vi "AudioTest.AudioTestUtil, Read Config.vi"(7 "File":path=path "c:/MTE/Audio Test/Config/Audio Util Config.ini", 8 "RtSetup":T1={"Play Device"="Utah", "Play Volume"=80.0, "DTMF Channel"=7, "Rec Device"="Jabra"} caption="Right Speaker Test Setup", 9 "LftSetup":T1={"Play Device"="Utah", "Play Volume"=80.0, "DTMF Channel"=4, "Rec Device"="Jabra"} caption="Left Speaker Test Setup", 10 "MicSetup":T1={"Play Device"="Jabra", "Play Volume"=60.0, "DTMF Channel"=1, "Rec Device"="Valve"} caption="Microphone Test Setup", 11 "ToneDur":dbl=0.3 caption="Tone Duration(s)") -> (0 "RtSetup Out":T1={"Play Device"="Utah", "Play Volume"=80.0, "DTMF Channel"=7, "Rec Device"="Jabra"} caption="Right Speaker Test Setup", 1 "LftSetup Out":T1={"Play Device"="Utah", "Play Volume"=80.0, "DTMF Channel"=4, "Rec Device"="Jabra"} caption="Left Speaker Test Setup", 2 "MicSetup Out":T1={"Play Device"="Jabra", "Play Volume"=60.0, "DTMF Channel"=1, "Rec Device"="Valve"} caption="Microphone Test Setup", 3 "ToneDur Out":dbl=0.3 caption="Tone Duration(s)", 4 "error out":errorcluster)   [LabVIEW 2018]
uses:
  <vilib>/Utility/config.llb/Read Key (Double).vi
  <vilib>/Utility/config.llb/Read Key (String).vi
  <vilib>/Utility/config.llb/Read Key (I32).vi
  <vilib>/Utility/config.llb/NI_LVConfig.lvlib
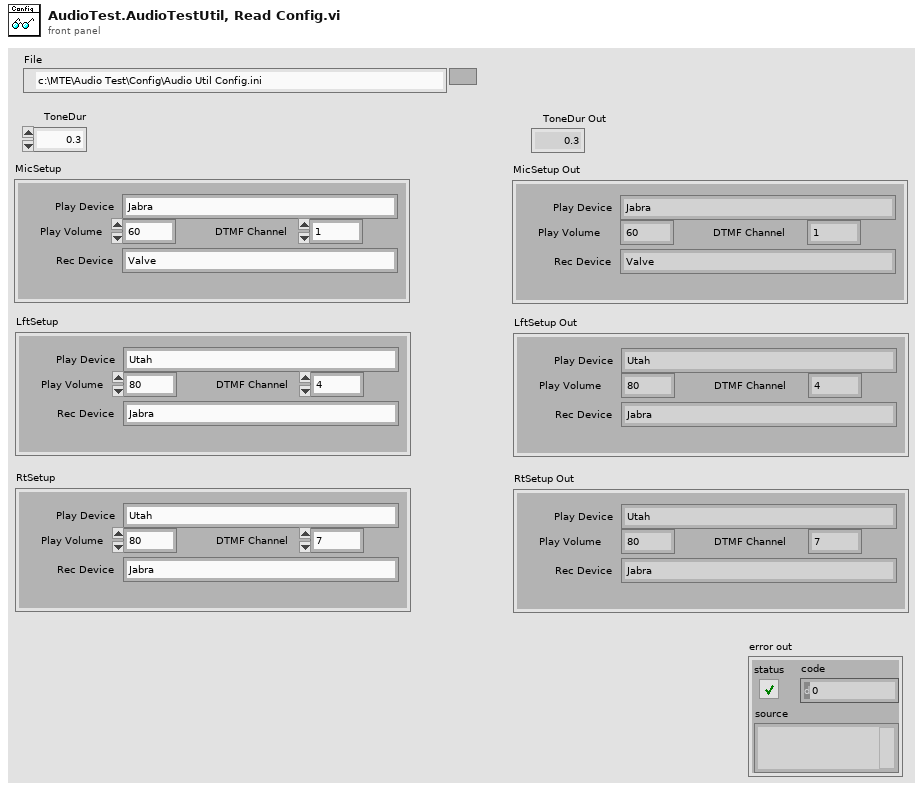
[diagram p1: front panel]
types:
  T1 = cluster{"Play Device":string, "Play Volume":dbl, "DTMF Channel":i32, "Rec Device":string}
  T2 = typedef "NI_LVConfig.lvlib/Config Data RefNum.ctl" = refnum<k1>
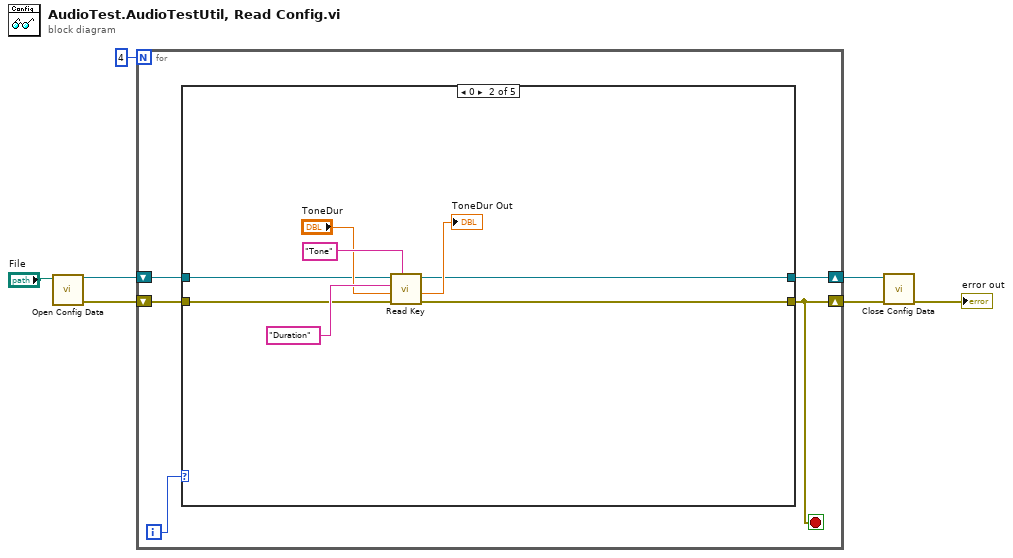
[diagram p0: block diagram]
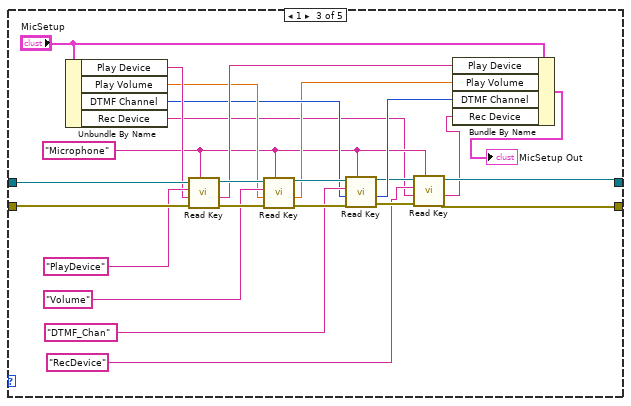
[diagram p3: hidden frame]
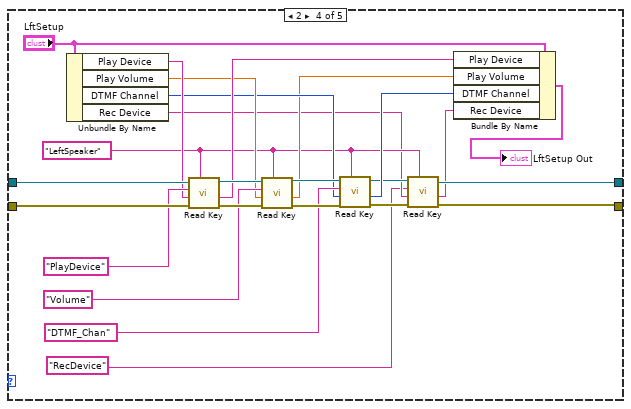
[diagram p4: hidden frame]
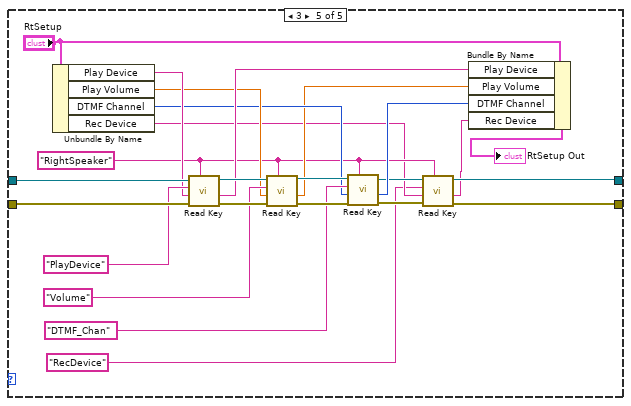
[diagram p5: hidden frame]
diagram:
  n1 = call <vilib>:"Open Config Data.vi"("configuration file path"="File") -> ("error out"=w6:errorcluster, "refnum"=w5:T2)  [unwired: 8 in, 1 out]
  n2 = for {
    N: 4 -> [_]
    shift-right: [w10] -> w3
    shift-left: w5 -> [w11]
    shift-right: [w9] -> w2
    shift-left: w6 -> [w12]
    i -> [w8]
    stop <- w9 stop-if-true
    n3 = case shown="0" w8 {
      tunnel: w12 -> [w13 w18 w46 w71 w96]
      tunnel: w11 -> [w14 w17 w47 w72 w97]
      tunnel: [w14 w16 w28 w52 w77] -> w10
      tunnel: [w13 w15 w27 w53 w78] -> w9
      frame Default {
      }
      frame 0 {
        n4 = call-poly <vilib>:"Read Key.vi"("section"="Tone", "error in (no error)"=w18, "default value"="ToneDur", "key"="Duration", "refnum"=w17) -> ("error out"=w15:errorcluster, "value"=→"ToneDur Out":dbl, "refnum out"=w16:T2)  [unwired: 3 in, 1 out]
      }
      frame 1 {
        w30 = "Microphone"
        n5 = Unbundle By Name("MicSetup") -> ("Play Device"=w36:string, "Play Volume"=w35:dbl, "DTMF Channel"=w34:i32, "Rec Device"=w24:string)
        n6 = call-poly <vilib>:"Read Key.vi"("section"=w30, "error in (no error)"=w46, "default value"=w36, "key"="PlayDevice", "refnum"=w47) -> ("error out"=w45:errorcluster, "value"=w37:string, "refnum out"=w42:T2)  [unwired: 3 in, 1 out]
        n7 = call-poly <vilib>:"Read Key.vi"("section"=w30, "error in (no error)"=w45, "default value"=w35, "key"="Volume", "refnum"=w42) -> ("error out"=w44:errorcluster, "value"=w32:dbl, "refnum out"=w43:T2)  [unwired: 3 in, 1 out]
        n8 = call-poly <vilib>:"Read Key.vi"("section"=w30, "error in (no error)"=w44, "default value"=w34, "key"="DTMF_Chan", "refnum"=w43) -> ("error out"=w26:errorcluster, "value"=w33:i32, "refnum out"=w29:T2)  [unwired: 3 in, 1 out]
        n9 = call-poly <vilib>:"Read Key.vi"("section"=w30, "error in (no error)"=w26, "default value"=w24, "key"="RecDevice", "refnum"=w29) -> ("error out"=w27:errorcluster, "value"=w23:string, "refnum out"=w28:T2)  [unwired: 3 in, 1 out]
        n10 = Bundle By Name(cluster="MicSetup", "Play Device"=w37, "Play Volume"=w32, "DTMF Channel"=w33, "Rec Device"=w23) -> (→"MicSetup Out":T1)
      }
      frame 2 {
        w51 = "LeftSpeaker"
        n11 = Unbundle By Name("LftSetup") -> ("Play Device"=w62:string, "Play Volume"=w61:dbl, "DTMF Channel"=w60:i32, "Rec Device"=w50:string)
        n12 = call-poly <vilib>:"Read Key.vi"("section"=w51, "error in (no error)"=w71, "default value"=w62, "key"="PlayDevice", "refnum"=w72) -> ("error out"=w70:errorcluster, "value"=w63:string, "refnum out"=w67:T2)  [unwired: 3 in, 1 out]
        n13 = call-poly <vilib>:"Read Key.vi"("section"=w51, "error in (no error)"=w70, "default value"=w61, "key"="Volume", "refnum"=w67) -> ("error out"=w69:errorcluster, "value"=w58:dbl, "refnum out"=w68:T2)  [unwired: 3 in, 1 out]
        n14 = call-poly <vilib>:"Read Key.vi"("section"=w51, "error in (no error)"=w69, "default value"=w60, "key"="DTMF_Chan", "refnum"=w68) -> ("error out"=w54:errorcluster, "value"=w59:i32, "refnum out"=w55:T2)  [unwired: 3 in, 1 out]
        n15 = call-poly <vilib>:"Read Key.vi"("section"=w51, "error in (no error)"=w54, "default value"=w50, "key"="RecDevice", "refnum"=w55) -> ("error out"=w53:errorcluster, "value"=w49:string, "refnum out"=w52:T2)  [unwired: 3 in, 1 out]
        n16 = Bundle By Name(cluster="LftSetup", "Play Device"=w63, "Play Volume"=w58, "DTMF Channel"=w59, "Rec Device"=w49) -> (→"LftSetup Out":T1)
      }
      frame 3 {
        w76 = "RightSpeaker"
        n17 = Unbundle By Name("RtSetup") -> ("Play Device"=w87:string, "Play Volume"=w86:dbl, "DTMF Channel"=w85:i32, "Rec Device"=w75:string)
        n18 = call-poly <vilib>:"Read Key.vi"("section"=w76, "error in (no error)"=w96, "default value"=w87, "key"="PlayDevice", "refnum"=w97) -> ("error out"=w95:errorcluster, "value"=w88:string, "refnum out"=w92:T2)  [unwired: 3 in, 1 out]
        n19 = call-poly <vilib>:"Read Key.vi"("section"=w76, "error in (no error)"=w95, "default value"=w86, "key"="Volume", "refnum"=w92) -> ("error out"=w94:errorcluster, "value"=w83:dbl, "refnum out"=w93:T2)  [unwired: 3 in, 1 out]
        n20 = call-poly <vilib>:"Read Key.vi"("section"=w76, "error in (no error)"=w94, "default value"=w85, "key"="DTMF_Chan", "refnum"=w93) -> ("error out"=w79:errorcluster, "value"=w84:i32, "refnum out"=w80:T2)  [unwired: 3 in, 1 out]
        n21 = call-poly <vilib>:"Read Key.vi"("section"=w76, "error in (no error)"=w79, "default value"=w75, "key"="RecDevice", "refnum"=w80) -> ("error out"=w78:errorcluster, "value"=w74:string, "refnum out"=w77:T2)  [unwired: 3 in, 1 out]
        n22 = Bundle By Name(cluster="RtSetup", "Play Device"=w88, "Play Volume"=w83, "DTMF Channel"=w84, "Rec Device"=w74) -> (→"RtSetup Out":T1)
      }
    }
  }
  n23 = call <vilib>:"Close Config Data.vi"("error in (no error)"=w2, "refnum"=w3) -> ("error out"=→"error out":errorcluster)  [unwired: 8 in, 1 out]
